vi "Read Write_Loop.vi"() -> ()   [LabVIEW 2020, in "NTV Read Write.lvlib"]
uses:
  NTV Read Write.lvlib
  AUTO 2023/Cluster_CMD_CMD_Data.ctl
  Shared Code/TypeDefs/ENUM_AutoSelect.ctl
  ENUM_SEN_State.ctl
  ENUM_SEN_Action.ctl
  41f29cb5-231b-4dac-ad95-cd6ae786e565.vi
  Utility/Global_STOP.vi
  AUTO 2023/Global_CMD_CMD_Data In.vi
  Global_SEN_Data Out.vi
  AUTO 2023/2023-Auto_CMD.lvlib
panel:
  out "Command Data Out":T1={"Auto Select"=enum."Drop mid dock and engage"}
  out "Cycle Time (S)":dbl format="%.3g"
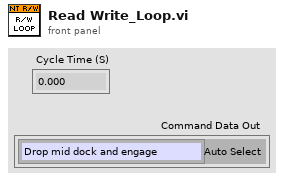
[diagram p1: front panel]
types:
  T1 = typedef "2023-Auto_CMD.lvlib/Cluster_CMD_CMD_Data.ctl" = cluster{"Auto Select":T2}
  T2 = typedef "ENUM_AutoSelect.ctl" = enum16{"Unknown", "Drop High Drive Straight", "Drop mid dock and engage", "Drop High dock and engage", "Drop Low dock and engage", "Manual", "Over and Rebalance", "Over and Dock"}
  T3 = typedef "NTV Read Write.lvlib/ENUM_SEN_State.ctl" = enum16{"Startup", "Exchanging Variables", "Shutdown"}
  T4 = typedef "NTV Read Write.lvlib/ENUM_SEN_Action.ctl" = enum16{"No Action", "Reset Time", "Read NT Variables", "Write NT Variables"}
  T5 = cluster{"State":T3, "Previous State":T3, "Current Time":timestamp, "Previous Time":timestamp, "Start Time":timestamp, "Target Time (ms)":u32, "Cycle Time(S)":dbl, "SEN Output DBL":dbl, "Read Enable":bool}
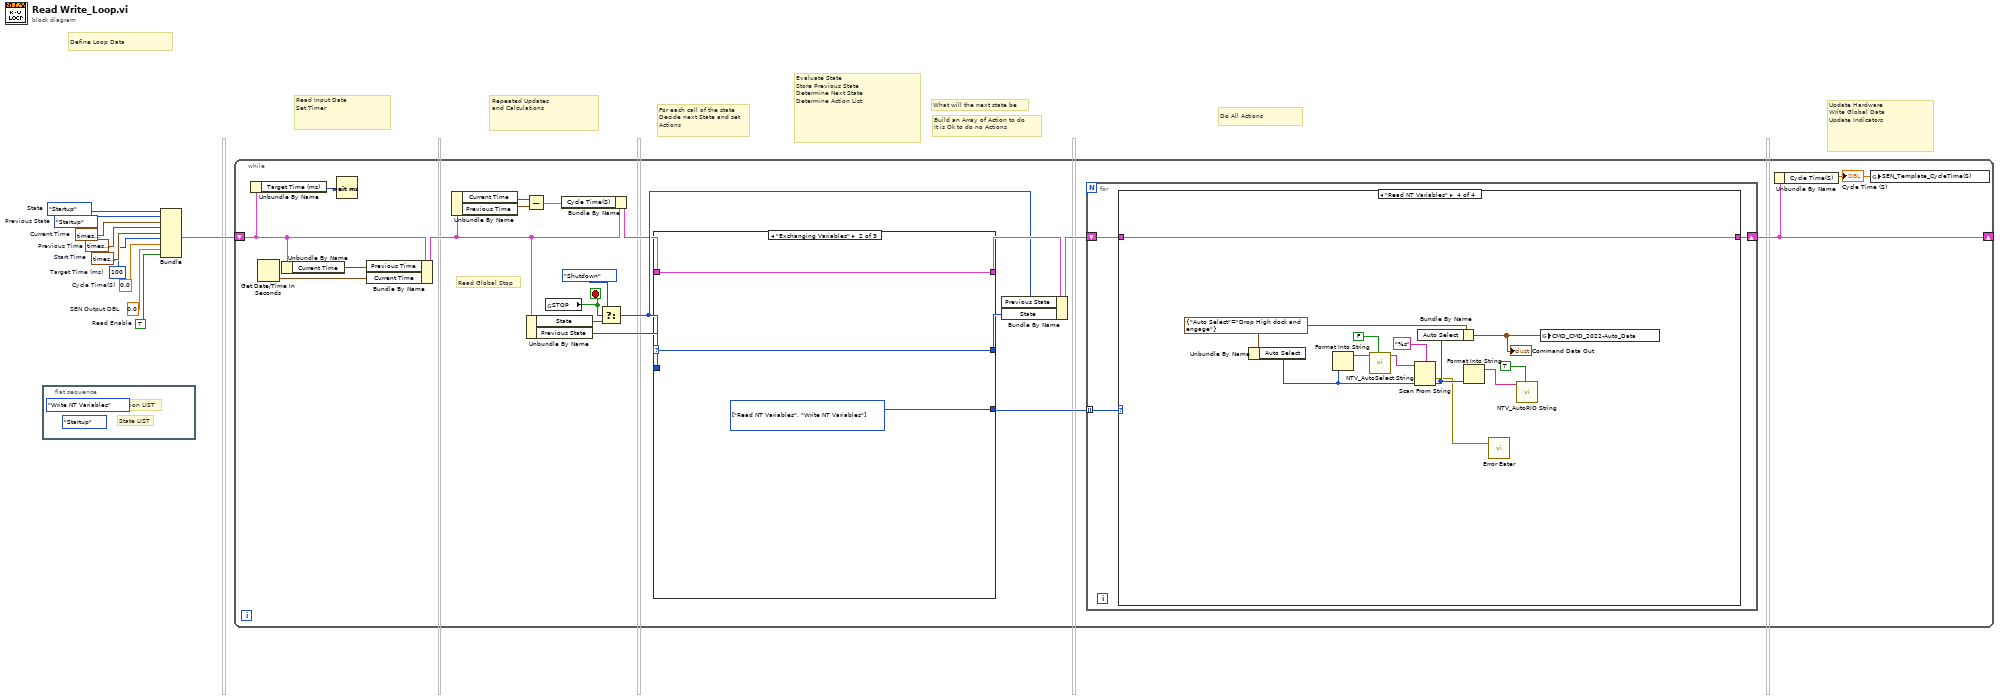
[diagram p0: block diagram]
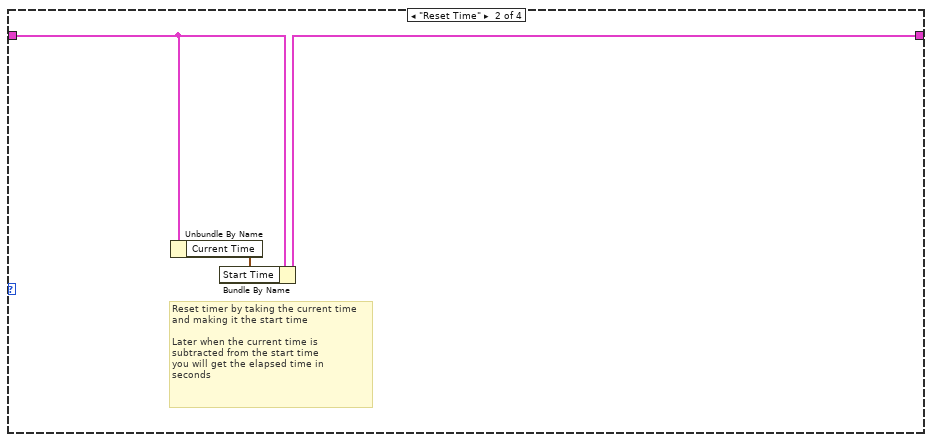
[diagram p3: hidden frame]
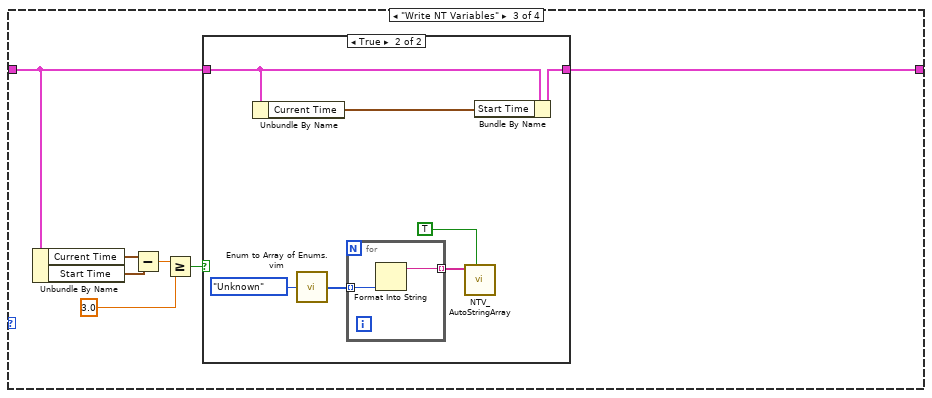
[diagram p4: hidden frame]
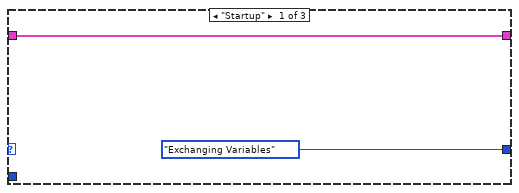
[diagram p6: hidden frame]
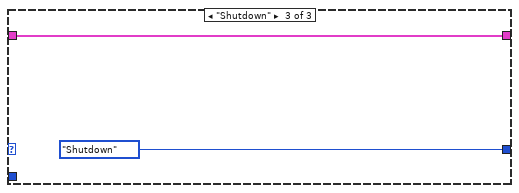
[diagram p7: hidden frame]
diagram:
  w2 = TRUE  # Read Enable
  w3 = 0.0  # Cycle Time(S)
  w4 = ENUM_SEN_State."Startup"  # Previous State
  w5 = timestamp(0 s since 1904-01-01)  # Previous Time
  w6 = u32 100  # Target Time (ms)
  w7 = 0.0  # SEN Output DBL
  w8 = timestamp(0 s since 1904-01-01)  # Start Time
  w9 = timestamp(0 s since 1904-01-01)  # Current Time
  w10 = ENUM_SEN_State."Startup"  # State
  # "Build an Array of Action to do\nIt is Ok to do no Actions"
  # "What will the next state be"
  # "For each call of the state\nDecide next State and set\nActions"
  # "Define Loop Data"
  # "Repeated Updates\nand Calculations"
  # "Read Input Data\nSet Timer"
  # "Evaluate State\nStore Previous State\nDetermine Next State\nDetermine Action List"
  # "Do All Actions"
  # "Update Hardware\nWrite Global Data\nUpdate Indicators"
  n1 = flat-sequence {
    frame #0 {
      (unwired) ENUM_SEN_State."Startup" ("State")
      (unwired) ENUM_SEN_Action."Write NT Variables" ("Action")
      # "State LIST"
      # "Action LIST"
    }
  }
  n2 = Bundle("State"=w10, "Previous State"=w4, "Current Time"=w9, "Previous Time"=w5, "Start Time"=w8, "Target Time (ms)"=w6, "Cycle Time(S)"=w3, "SEN Output DBL"=w7, "Read Enable"=w2) -> (w1:T5)  [unwired: 1 in]
  n3 = while {
    shift-right: [w11] -> _
    shift-left: w1 -> [w21]
    stop <- w26 stop-if-true
    # "Read Global Stop"
    n4 = Unbundle By Name(w21) -> ("Target Time (ms)"=w23:u32)
    n5 = Get Date/Time In Seconds() -> (seconds since 1Jan1904=w30:timestamp)
    n6 = Unbundle By Name(w21) -> ("Current Time"=w22:timestamp)
    n7 = Wait (ms)(milliseconds to wait=w23) -> ()  [unwired: 1 out]
    n8 = Bundle By Name(cluster=w21, "Previous Time"=w22, "Current Time"=w30) -> (w16:T5)
    n9 = Unbundle By Name(w16) -> ("Current Time"=w17:timestamp, "Previous Time"=w18:timestamp)
    n10 = Subtract(x=w17, y=w18) -> (x-y=w14:dbl)
    n11 = Unbundle By Name(w16) -> ("State"=w24:T3, "Previous State"=w20:T3)
    n12 = global read "Global_STOP.vi" "STOP"() -> (w26:bool)
    n13 = Bundle By Name(cluster=w16, "Cycle Time(S)"=w14) -> (w15:T5)
    n14 = Select(t=ENUM_SEN_State."Shutdown" ("State"), s=w26, f=w24) -> (s? t:f=w19:T3)
    n15 = case shown="\"Exchanging Variables\"" w19 {
      selector: w19 -> [_ w69 _]
      tunnel: w15 -> [w68 w71 w73]
      tunnel: [w68 w71 w73] -> w28
      tunnel: [ENUM_SEN_State."Exchanging Variables" ("State") w69 ENUM_SEN_State."Shutdown" ("State")] -> w27
      tunnel: [_ w70 _] -> w13
      tunnel: w20 -> [_ _ _]
      frame "Startup" {
      }
      frame "Exchanging Variables" {
        w70 = T4[] [enum."Read NT Variables", enum."Write NT Variables"] items=["No Action", "Reset Time", "Read NT Variables", "Write NT Variables"] ("Actions")
      }
      frame "Shutdown" {
      }
    }
    n16 = Bundle By Name(cluster=w28, "Previous State"=w19, "State"=w27) -> (w29:T5)
    n17 = for {
      tunnel: w13 -> [w33] mode=indexing
      shift-right: [w32] -> w11
      shift-left: w29 -> [w31]
      n18 = case shown="\"Read NT Variables\"" w33 {
        tunnel: w31 -> [w34 w37 w44 w66]
        tunnel: [w34 w36 w43 w66] -> w32
        frame "No Action" {
        }
        frame "Reset Time" {
          # "Reset timer by taking the current time\nand making it the start time\n\nLater when the current time is \nsubtracted from the start time\nyou will get the elapsed time in \nseconds"
          n19 = Unbundle By Name(w37) -> ("Current Time"=w35:timestamp)
          n20 = Bundle By Name(cluster=w37, "Start Time"=w35) -> (w36:T5)
        }
        frame "Write NT Variables" {
          n21 = Unbundle By Name(w44) -> ("Current Time"=w42:timestamp, "Start Time"=w41:timestamp)
          n22 = Subtract(x=w42, y=w41) -> (x-y=w40:dbl)
          n23 = Greater Or Equal?(x=w40, y=3.0) -> (x >= y?=w38:bool)
          n24 = case shown="True" w38 {
            tunnel: w44 -> [w45 w47]
            tunnel: [w45 w48] -> w43
            frame False {
            }
            frame True {
              n25 = Unbundle By Name(w47) -> ("Current Time"=w46:timestamp)
              n26 = call "Enum to Array of Enums.vim"("enum"=ENUM_AutoSelect."Unknown" ("Auto Select")) -> ("array of enums"=w51:T2[])
              n27 = for {
                tunnel: w51 -> [w54] mode=indexing
                tunnel: [w53] -> w50 mode=indexing
                n28 = Format Into String(w54) -> (resulting string=w53:string)  [unwired: 3 in, 1 out]
              }
              n29 = call "NTV_AutoStringArray.vi"("Read(f) Write(t)"=TRUE, "Array"=w50) -> ()  [unwired: 9 in, 1 out]
              n30 = Bundle By Name(cluster=w47, "Start Time"=w46) -> (w48:T5)
            }
          }
        }
        frame "Read NT Variables" {
          w63 = T1 {"Auto Select"=enum."Drop High dock and engage"} ("CMD_CMD_2022-Auto_Data")
          n31 = Unbundle By Name(w63) -> ("Auto Select"=w61:T2)
          n32 = Format Into String(w61) -> (resulting string=w62:string)  [unwired: 3 in, 1 out]
          n33 = call "NTV_AutoSelect String.vi"("Read(f) Write(t)"=FALSE, "Auto RIO"=w62) -> ("Auto RIO"=w59:string)  [unwired: 9 in]
          n34 = Scan From String(format string="%s", input string=w59, default 1=w61) -> (error out=w55:errorcluster, output 1=w58:T2)  [unwired: 2 in, 2 out]
          n35 = Bundle By Name(cluster=w63, "Auto Select"=w58) -> (w64:T1)
          "Command Data Out" <- w64
          n36 = Format Into String(w58) -> (resulting string=w57:string)  [unwired: 3 in, 1 out]
          n37 = call "Error Eater.vi"("error in (no error)"=w55) -> ()  [unwired: 2 in]
          n38 = call "NTV_AutoRIO String.vi"("Read(f) Write(t)"=TRUE, "Auto RIO"=w57) -> ()  [unwired: 9 in, 1 out]
          n39 = global write "Global_CMD_CMD_Data In.vi" "CMD_CMD_2022-Auto_Data"(w64) -> ()
        }
      }
    }
    n40 = Unbundle By Name(w11) -> ("Cycle Time(S)"=w12:dbl)
    "Cycle Time (S)" <- w12
    n41 = global write "Global_SEN_Data Out.vi" "SEN_Template_CycleTime(S)"(w12) -> ()
  }
